vi "ControlRoom-RT.vi"() -> ()   [LabVIEW 2016]
uses:
  <vilib>/rvi/interface/nirviOpenFPGA/nirviOpenFPGA.xnode
  <vilib>/rvi/interface/nirviReadWriteControl/nirviReadWriteControl.xnode
  Common-Control/Beamline sections/Control Room/ControlRoom-FPGA.vi
  <vilib>/Utility/error.llb/Error Cluster From Error Code.vi
  <vilib>/rvi/errors/niLvFpgaAdjustHostInterfaceError.vi
  <vilib>/Platform/TimedLoop/XDataNode/XDataNode.xnode
  <vilib>/Platform/TimedLoop/XDataNode/nitl_modes.ctl
  <vilib>/Platform/TimedLoop/XDataNode/XDNodeRunTimeDep.lvlib
  <vilib>/Platform/TimedLoop/XDataNode/wakeup.ctl
  <vilib>/Platform/TimedLoop/XDataNode/timing_clust.ctl
  NiFpgaLv.dll
  FPGA Bitfiles/PRIMEControl2017_FPGATarget6_ControlRoom-FPGA_EInbnQLA0MM.lvbitx
  <vilib>/FPGAPlugInAG/cRIO-9074/niLvFpga_Open_cRIO-9074.vi
panel:
  in  "Tab Control":enum32{"High Voltage", "Errors"}(tab)
  out "Terminal voltage":dbl format="%_3g"
  out "Corona":dbl format="%_3g"
  out "Grid":dbl format="%_3g"
  out "He Sup":dbl format="%_3g"
  out "He Ind":dbl format="%_3g"
  out "He chain":dbl format="%_3g"
  out "He column":dbl format="%_3g"
  out "Le column":dbl format="%_3g"
  out "Le chain":dbl format="%_3g"
  out "Le Ind":dbl format="%_3g"
  out "Le Sup":dbl format="%_3g"
  out "ControlRoom-cRIO error":errorcluster
  out "Readback loop error":errorcluster
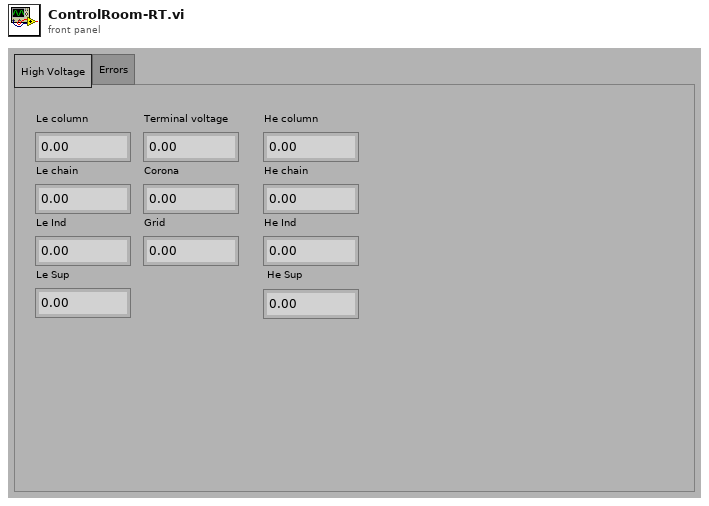
[diagram p1: front panel]
types:
  T1 = typedef "XDNodeRunTimeDep.lvlib/timing_clust.ctl" = cluster{"Expected End [f-1]":u64, "Actual End [f-1]":u64, "Finished Late? [f-1]":bool, "Expected End [i-1]":u64, "Actual End [i-1]":u64, "Finished Late? [i-1]":bool, "Expected Start [i]":u64, "Actual Start [i]":u64, "Expected Start [f]":u64, "Actual Start [f]":u64, "Source Name":string, "Structure Name":string, "Period":i64, "Deadline":i64, "Offset":i64, "Start":i64, "Priority":i32, "Timeout":i32, "Mode":T2, "Wakeup Reason":T3, "Error":errorcluster, "Source Type":string, "Secondary Source Type":string, "Global End Time":u64, "Global Start Time":u64, "Frame Duration":u64, "Iteration Duration":u64, "Assigned CPU":i32, "I/O Scan Engine Mode":u32}
  T2 = typedef "XDNodeRunTimeDep.lvlib/nitl_modes.ctl" = enum32{"No Change", "Process missed periods, maintain original phase", "Discard missed periods, maintain original phase", "Process missed periods, ignore original phase", "Discard missed periods, ignore original phase"}
  T3 = typedef "XDNodeRunTimeDep.lvlib/wakeup.ctl" = enum32{"Normal", "Aborted", "Asynchronous wakeup", "Timing source error", "Timed loop error", "Timeout"}
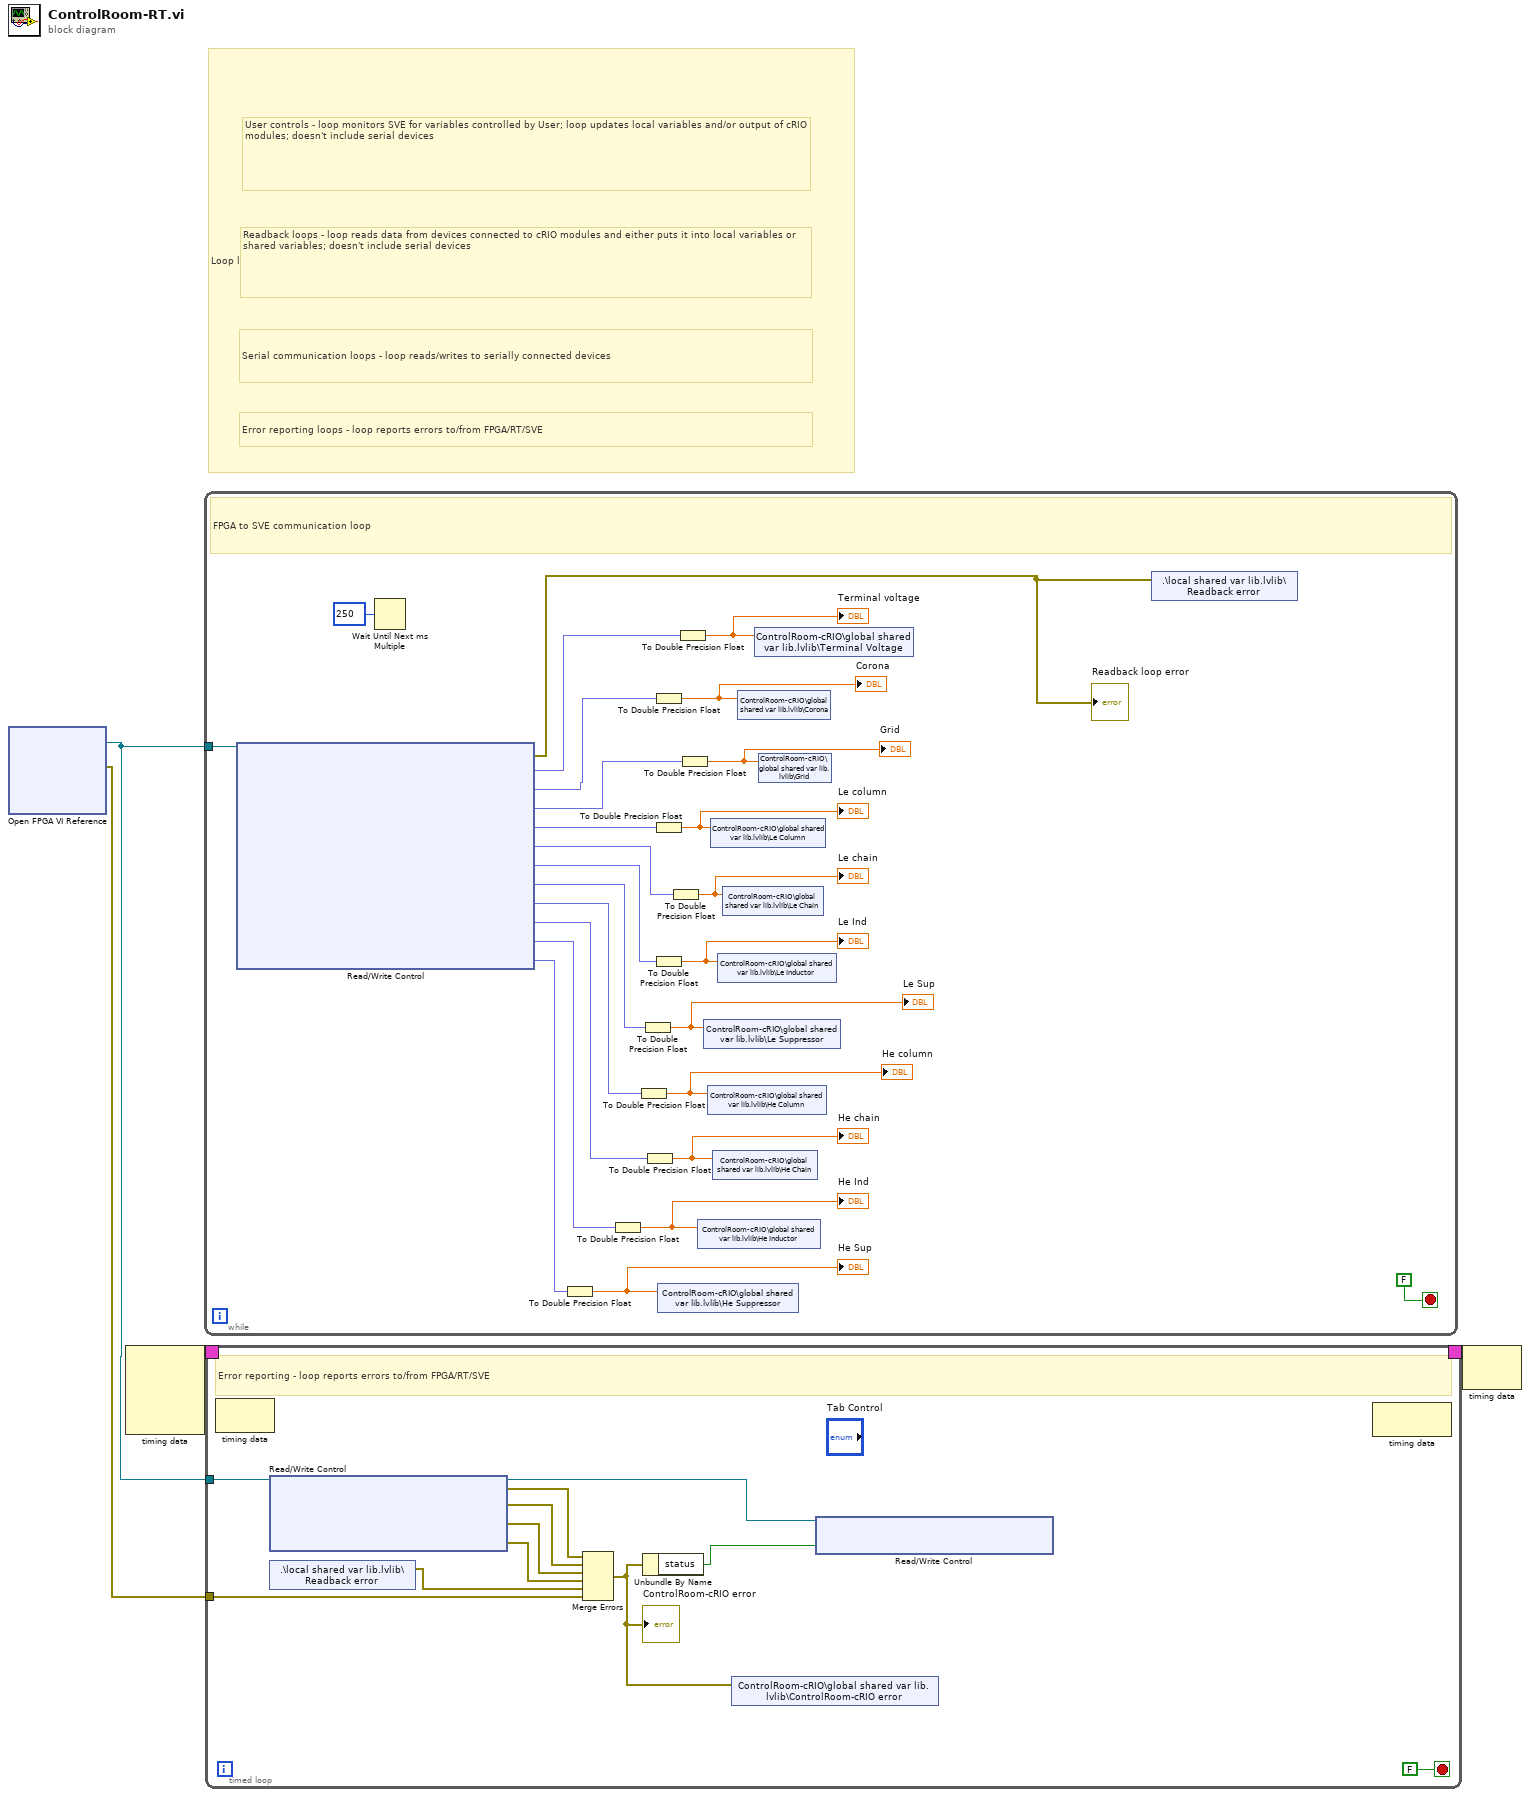
[diagram p0: block diagram]
diagram:
  # "Error reporting loops - loop reports errors to/from FPGA/RT/SVE"
  # "Serial communication loops - loop reads/writes to serially connected devices"
  # "Readback loops - loop reads data from devices connected to cRIO modules and either puts it into local variables or shared variables; doesn't include serial devices"
  # "User controls - loop monitors SVE for variables controlled by User; loop updates local variables and/or output of cRIO modules; doesn't include serial devices"
  # "Loop legend - loops are color coded by responsibility"
  n1 = xnode "Open FPGA VI Reference"() -> ("FPGA VI Reference Out"=w2:refnum<k20>, "error out"=w1:errorcluster)  [unwired: 2 in]
  n2 = node-c288() -> (w4:T1)  [unwired: 4 in]
  n3 = while {
    tunnel: w2 -> [w29]
    stop <- FALSE stop-if-true
    # "FPGA to SVE communication loop"
    n4 = xnode "Read/Write Control"("FPGA VI Reference In"=w29) -> ("error out"=w6:errorcluster, "Terminal Readbacks.GVM Voltage"=w28:fxp<+/-,26,5>, "Terminal Readbacks.Corona Probe Current"=w27:fxp<+/-,26,5>, "Terminal Readbacks.Grid Voltage"=w26:fxp<+/-,26,5>, "LE Readbacks.Column Current"=w25:fxp<+/-,26,5>, "LE Readbacks.Chain Current"=w24:fxp<+/-,26,5>, "LE Readbacks.Inductor"=w23:fxp<+/-,26,5>, "LE Readbacks.Suppressor"=w22:fxp<+/-,26,5>, "HE Readbacks.Column Current"=w21:fxp<+/-,26,5>, "HE Readbacks.Chain Current"=w20:fxp<+/-,26,5>, "HE Readbacks.Inductor"=w19:fxp<+/-,26,5>, "HE Readbacks.Suppressor"=w18:fxp<+/-,26,5>)  [unwired: 1 in, 1 out]
    "Readback loop error" <- w6
    n5 = Wait Until Next ms Multiple(millisecond multiple=u32 250) -> ()  [unwired: 1 out]
    n6 = To Double Precision Float(number=w18) -> (double precision float=w17:dbl)
    "He Sup" <- w17
    n7 = To Double Precision Float(number=w19) -> (double precision float=w16:dbl)
    "He Ind" <- w16
    n8 = To Double Precision Float(number=w21) -> (double precision float=w14:dbl)
    "He column" <- w14
    n9 = To Double Precision Float(number=w22) -> (double precision float=w13:dbl)
    "Le Sup" <- w13
    n10 = To Double Precision Float(number=w20) -> (double precision float=w15:dbl)
    "He chain" <- w15
    n11 = To Double Precision Float(number=w27) -> (double precision float=w11:dbl)
    "Corona" <- w11
    n12 = To Double Precision Float(number=w25) -> (double precision float=w9:dbl)
    "Le column" <- w9
    n13 = To Double Precision Float(number=w23) -> (double precision float=w7:dbl)
    "Le Ind" <- w7
    n14 = shared-variable "ControlRoom-cRIO\\global shared var lib.lvlib\\He Suppressor"(w17) -> ()  [unwired: 1 in, 1 out]
    n15 = To Double Precision Float(number=w24) -> (double precision float=w8:dbl)
    "Le chain" <- w8
    n16 = To Double Precision Float(number=w28) -> (double precision float=w12:dbl)
    "Terminal voltage" <- w12
    n17 = To Double Precision Float(number=w26) -> (double precision float=w10:dbl)
    "Grid" <- w10
    n18 = shared-variable "ControlRoom-cRIO\\global shared var lib.lvlib\\He Inductor"(w16) -> ()  [unwired: 1 in, 1 out]
    n19 = shared-variable "ControlRoom-cRIO\\global shared var lib.lvlib\\Le Suppressor"(w13) -> ()  [unwired: 1 in, 1 out]
    n20 = shared-variable "ControlRoom-cRIO\\global shared var lib.lvlib\\He Column"(w14) -> ()  [unwired: 1 in, 1 out]
    n21 = shared-variable "ControlRoom-cRIO\\global shared var lib.lvlib\\Le Column"(w9) -> ()  [unwired: 1 in, 1 out]
    n22 = shared-variable "ControlRoom-cRIO\\global shared var lib.lvlib\\He Chain"(w15) -> ()  [unwired: 1 in, 1 out]
    n23 = shared-variable "ControlRoom-cRIO\\global shared var lib.lvlib\\Le Inductor"(w7) -> ()  [unwired: 1 in, 1 out]
    n24 = shared-variable "ControlRoom-cRIO\\global shared var lib.lvlib\\Le Chain"(w8) -> ()  [unwired: 1 in, 1 out]
    n25 = shared-variable "ControlRoom-cRIO\\global shared var lib.lvlib\\Corona"(w11) -> ()  [unwired: 1 in, 1 out]
    n26 = shared-variable "ControlRoom-cRIO\\global shared var lib.lvlib\\Terminal Voltage"(w12) -> ()  [unwired: 1 in, 1 out]
    n27 = shared-variable "ControlRoom-cRIO\\global shared var lib.lvlib\\Grid"(w10) -> ()  [unwired: 1 in, 1 out]
    n28 = shared-variable ".\\local shared var lib.lvlib\\Readback error"(w6) -> ()  [unwired: 1 in, 1 out]
  }
  n29 = timed-loop {
    timing: w4 -> [_]
    timing-out: [_] -> w3
    tunnel: w2 -> [w39]
    tunnel: w1 -> [w31]
    stop <- FALSE stop-if-true
    # "Error reporting - loop reports errors to/from FPGA/RT/SVE"
    n30 = node-c288() -> ()  [unwired: 1 in, 1 out]
    n31 = xnode "Read/Write Control"("FPGA VI Reference In"=w39) -> ("FPGA VI Reference Out"=w38:refnum<k20>, "error out"=w37:errorcluster, "Terminal error"=w36:errorcluster, "HE error"=w35:errorcluster, "LE error"=w34:errorcluster)  [unwired: 1 in]
    n32 = shared-variable ".\\local shared var lib.lvlib\\Readback error"() -> (w32:errorcluster)  [unwired: 1 in, 1 out]
    n33 = Merge Errors(w37, w36, w35, w34, w32, w31) -> (w40:errorcluster)
    "ControlRoom-cRIO error" <- w40
    n34 = Unbundle By Name(w40) -> ("status"=w41:bool)
    n35 = shared-variable "ControlRoom-cRIO\\global shared var lib.lvlib\\ControlRoom-cRIO error"(w40) -> ()  [unwired: 1 in, 1 out]
    n36 = xnode "Read/Write Control"("FPGA VI Reference In"=w38, "RT error"=w41) -> ()  [unwired: 1 in, 2 out]
    n37 = node-c288() -> ()  [unwired: 1 in, 1 out]
  }
  n38 = node-c288(w3) -> ()  [unwired: 1 out]
